vi "ITC503 write A.vi"(8 "error in (no error) 2":errorcluster, 10 "write buffer 2":string, 11 "VISA resource name 2":refnum<visa-resource-name>) -> (0 "error out 2":errorcluster, 1 "VISA resource name out 2":refnum<visa-resource-name>, 2 "read buffer 2":string, 3 "Numeric":dbl)   [LabVIEW 2010]
panel:
  in  "write buffer":string
  out "read buffer":string
  out "VISA resource name out":refnum<visa-resource-name>
  out "error out":errorcluster
  in  "error in (no error)":errorcluster
  in  "VISA resource name":refnum<visa-resource-name>
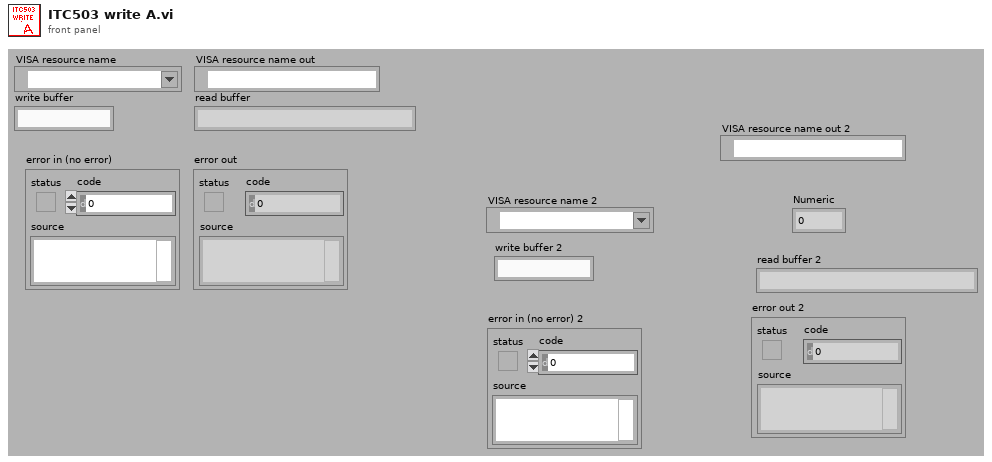
[diagram p1: front panel]
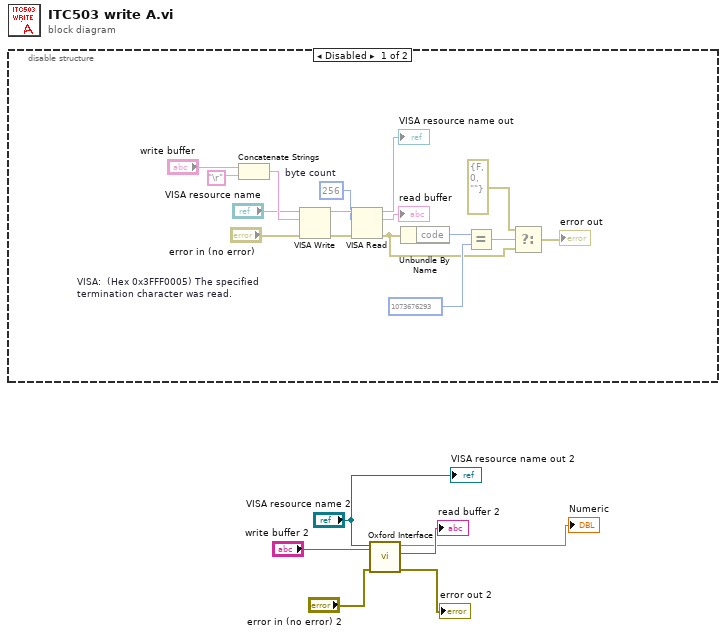
[diagram p0: block diagram]
diagram:
  n1 = disable-structure shown="Disabled" {
    frame Disabled {
      w13 = 1073676293  # VISA:  (Hex 0x3FFF0005) The specified termination character was read.
      w20 = u32 256  # byte count
      n2 = Concatenate Strings("write buffer", "\r") -> (w16:string)
      n3 = VISA Write(VISA resource name="VISA resource name", write buffer=w16, error in (no error)="error in (no error)") -> (VISA resource name out=w21:refnum<visa-resource-name>, error out=w22:errorcluster)  [unwired: 1 out]
      n4 = VISA Read(VISA resource name=w21, byte count=w20, error in (no error)=w22) -> (VISA resource name out=→"VISA resource name out":refnum<visa-resource-name>, read buffer=→"read buffer":string, error out=w11:errorcluster)  [unwired: 1 out]
      n5 = Unbundle By Name(w11) -> ("code"=w14:i32)
      n6 = Equal?(x=w14, y=w13) -> (x = y?=w10:bool)
      n7 = Select(t=errorcluster {"status"=FALSE, "code"=0, "source"=""}, s=w10, f=w11) -> (s? t:f=→"error out":errorcluster)
    }
    frame Enabled {
    }
  }
  n8 = call "Oxford Interface.vi"("error in (no error)"="error in (no error) 2", "Command"="write buffer 2", "Address"="VISA resource name 2") -> ("error out"=→"error out 2":errorcluster, "Reply"=→"read buffer 2":string, "Numeric reply"=→"Numeric":dbl)  [unwired: 6 out]
  "VISA resource name out 2" <- "VISA resource name 2"
